vi "Asylum_GetRange.vi"(8 "error in (no error)":errorcluster, 10 "parameterName":string, 11 "Application In":refnum<k7>) -> (0 "error out":errorcluster, 2 "Range":string, 3 "Application Out":refnum<k7>)   [LabVIEW 2019]
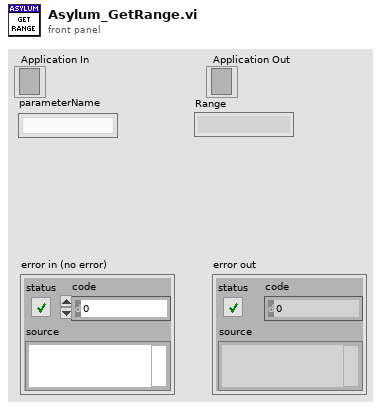
[diagram p1: front panel]
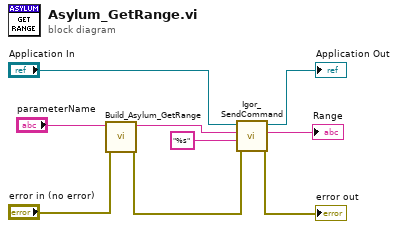
[diagram p0: block diagram]
diagram:
  n1 = call "Build_Asylum_GetRange.vi"("error in (no error)"="error in (no error)", "parameterName"="parameterName") -> ("error out"=w9:errorcluster, "Command"=w7:string)  [unwired: 8 in]
  n2 = call <userlib>:"Igor_SendCommand.vi"("error in (no error)"=w9, "Format"="%s", "command"=w7, "Application In"="Application In") -> ("error out"=→"error out":errorcluster, "results"=→"Range":string, "Application Out"=→"Application Out":refnum<k7>)  [unwired: 4 in, 1 out]
